vi "Global Variables.vi"() -> ()   [LabVIEW 2018]
panel:
  in  "Lab Configuration Path":path=path "X:/Lab Configuration"
  in  "Repository Path":path=path "C:/Users/bowenm/Documents/GitHub/MHDlab"
  in  "Data folder":path=path "F:/Data/Raw Data"
  in  "Global File Information":T1={"Project"=2, "SubFolder"="Test", "Filename (Meas. Description)"="None", "Measurement index"=0} {"Project" items=["UnspecifiedProj,Default unspecified project", "Proj_VaporTubes,Photoionization of Alkali Metal Vapor tubes", "Proj_H2DT,", "Proj_HVOF_PI,Photoionization in HVOF jet"]}
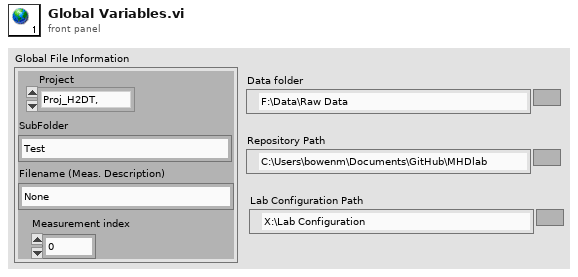
[diagram p1: front panel]
types:
  T1 = cluster{"Project":u16, "SubFolder":string, "Filename (Meas. Description)":string, "Measurement index":i32}
diagram:
